vi "WFDC Display Cam Image.vi"(0 "Image Ref":T1, 11 "Display?":bool) -> ()   [LabVIEW 2020]
uses:
  <vilib>/vision/Image Controls.llb/IMAQ Image.ctl
panel:
  out "Error Out":errorcluster
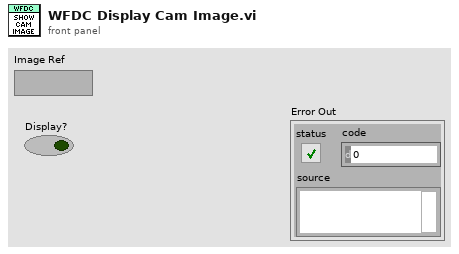
[diagram p1: front panel]
types:
  T1 = typedef "IMAQ Image.ctl" = refnum<image>
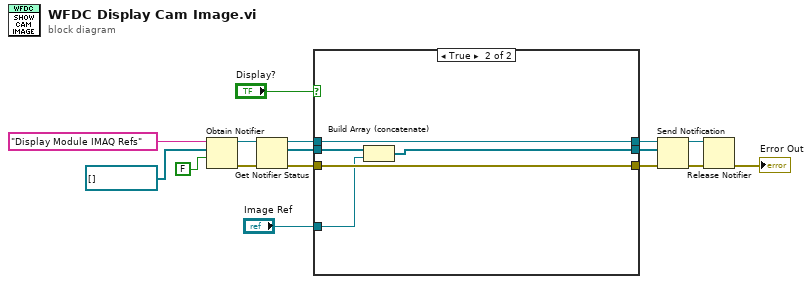
[diagram p0: block diagram]
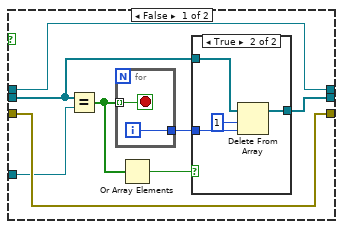
[diagram p2: hidden frame]
diagram:
  n1 = Obtain Notifier(name (unnamed)="Display Module IMAQ Refs", notification data type=T1[] [], create if not found? (T)=FALSE) -> (notifier out=w10:refnum<notifier>, error out=w9:errorcluster)  [unwired: 1 in, 1 out]
  n2 = Get Notifier Status(notifier=w10, error in (no error)=w9) -> (notifier out=w11:refnum<notifier>, current notification=w13:T1[], error out=w12:errorcluster)  [unwired: 2 out]
  n3 = case shown="True" "Display?" {
    tunnel: w11 -> [w24 w34]
    tunnel: w12 -> [w18 w33]
    tunnel: w13 -> [w20 w36]
    tunnel: [w19 w35] -> w16
    tunnel: [w24 w34] -> w14
    tunnel: [w18 w33] -> w15
    tunnel: "Image Ref" -> [w17 w32]
    frame False {
      n4 = Equal?(x=w20, y=w17) -> (x = y?=w23:bool[])
      n5 = for {
        tunnel: w23 -> [w31] mode=indexing
        tunnel: [w30] -> w21
        i -> [w30]
        stop <- w31 stop-if-true
      }
      n6 = Or Array Elements(Boolean array=w23) -> (logical OR=w22:bool)
      n7 = case shown="True" w22 {
        tunnel: w21 -> [_ w28]
        tunnel: w20 -> [w25 w27]
        tunnel: [w25 w26] -> w19
        frame False {
        }
        frame True {
          n8 = Delete From Array(array=w27, length=1, index=w28) -> (array with subset deleted=w26:T1[])  [unwired: 1 out]
        }
      }
    }
    frame True {
      n9 = Build Array (concatenate)(w36, w32) -> (w35:T1[])
    }
  }
  n10 = Send Notification(notification=w16, notifier=w14, error in (no error)=w15) -> (notifier out=w8:refnum<notifier>, error out=w7:errorcluster)
  n11 = Release Notifier(notifier=w8, error in (no error)=w7) -> (error out=→"Error Out":errorcluster)  [unwired: 1 in, 2 out]
